vi "svx_Colormap X Y to Map.vi"(5 "Plot area":T1, 7 "Range":T2, 11 "cordinate":cluster{"x":dbl, "y":dbl}) -> (0 "In?":bool, 3 "Map":cluster{"x":i16, "y":i16})   [LabVIEW 2017, in "SVX Colormap.xctl"]
uses:
  <vilib>/addons/_XControls/Colormap/SVX Colormap.xctl
  <vilib>/Utility/miscctls.llb/LVBoundsTypeDef.ctl
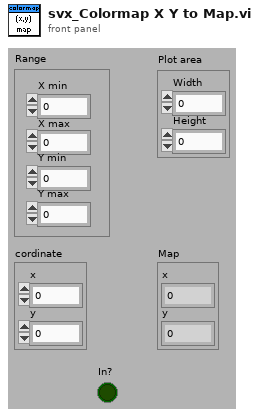
[diagram p1: front panel]
types:
  T1 = typedef "LVBoundsTypeDef.ctl" = cluster{"Width":u32, "Height":u32}
  T2 = cluster{"X min":dbl, "X max":dbl, "Y min":dbl, "Y max":dbl}
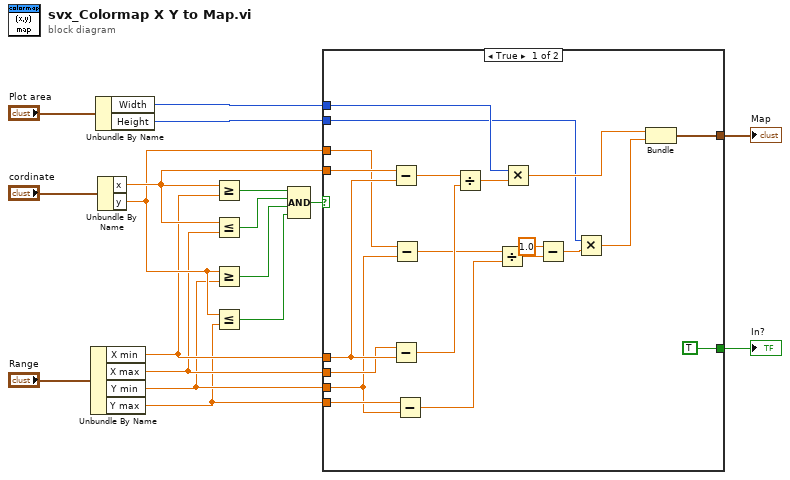
[diagram p0: block diagram]
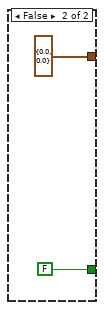
[diagram p2: hidden frame]
diagram:
  n1 = Unbundle By Name("Range") -> ("X min"=w5:dbl, "X max"=w4:dbl, "Y min"=w3:dbl, "Y max"=w2:dbl)
  n2 = Unbundle By Name("Plot area") -> ("Width"=w9:u32, "Height"=w8:u32)
  n3 = Unbundle By Name("cordinate") -> ("x"=w7:dbl, "y"=w6:dbl)
  n4 = Greater Or Equal?(x=w7, y=w5) -> (x >= y?=w16:bool)
  n5 = Less Or Equal?(x=w7, y=w4) -> (x <= y?=w15:bool)
  n6 = Greater Or Equal?(x=w6, y=w3) -> (x >= y?=w14:bool)
  n7 = Less Or Equal?(x=w6, y=w2) -> (x <= y?=w13:bool)
  n8 = Compound Arithmetic op=AND(w16, w15, w14, w13) -> (w12:bool)
  n9 = case shown="True" w12 {
    tunnel: [TRUE ("In?") FALSE ("In?")] -> w11
    tunnel: w9 -> [w32 _]
    tunnel: w8 -> [w20 _]
    tunnel: w7 -> [w37 _]
    tunnel: w6 -> [w29 _]
    tunnel: w5 -> [w36 _]
    tunnel: w4 -> [w35 _]
    tunnel: w3 -> [w26 _]
    tunnel: w2 -> [w27 _]
    tunnel: [w30 cluster{dbl, dbl} {0.0, 0.0}] -> w1
    frame True {
      n10 = Subtract(x=w37, y=w36) -> (x-y=w34:dbl)
      n11 = Subtract(x=w35, y=w36) -> (x-y=w28:dbl)
      n12 = Subtract(x=w29, y=w26) -> (x-y=w25:dbl)
      n13 = Subtract(x=w27, y=w26) -> (x-y=w24:dbl)
      n14 = Divide(x=w34, y=w28) -> (x/y=w33:dbl)
      n15 = Divide(x=w25, y=w24) -> (x/y=w23:dbl)
      n16 = Multiply(x=w32, y=w33) -> (x*y=w31:dbl)
      n17 = Subtract(x=1.0, y=w23) -> (x-y=w21:dbl)
      n18 = Multiply(x=w20, y=w21) -> (x*y=w19:dbl)
      n19 = Bundle(w31, w19) -> (w30:cluster{dbl, dbl})  [unwired: 1 in]
    }
    frame False {
    }
  }
  "In?" <- w11
  "Map" <- w1
